vi "101_VI_Analysis_G-CLI.vi"() -> ()   [LabVIEW 2023]
doc: "This example uses the advanced VI Analyzer VIs to perform an analysis on an LLB of VIs. The \"New Task\" VI uses preset test settings loaded from a CFG file that was created from the VI Analyzer user interface. Certain advanced VIs are used to perform tasks like adding an LLB to the analysis, removing a single VI from the analysis, removing certain tests from the analysis, and modifying a configuration value on one test. Once the analysis performed by \"VIAn Run.vi\" is complete, the \"VIAn Easy Report.vi\" saves the analysis results to an HTML report."
uses:
  <vilib>/addons/analyzer/NI_VIAnalyzerTKVIs.lvlib
  <vilib>/Wiresmith Technology/G CLI/CLI Class/CLI.lvclass
panel:
  out "Custom Parameters":string[](array[string])
  out "VI in Analysis":string
  out "Analysis Progress":dbl(slide) scale=0.0..100.0
  out "Tests Run":string[](array[string])
  out "VIs Tested":path[](array[path])
  # "Overview: Demonstrates the use of the VI Analyzer and VI Analyzer Utility VIs to customize a programmatic analysis.\nRequirements: VI Analyzer Toolkit\nInstructions:\nRun the VI."
  # "Exclude these tests from the VI Analyzer Task."
  # "Set these tests to have 10 maximum failures for the VI Analyzer Task."
  # "Remove the top-level placeholder VI from the analysis."
  # "Disable the option on the \"VI Documentation\" test to analyze control descriptions."
  # "Show the progress of the analysis."
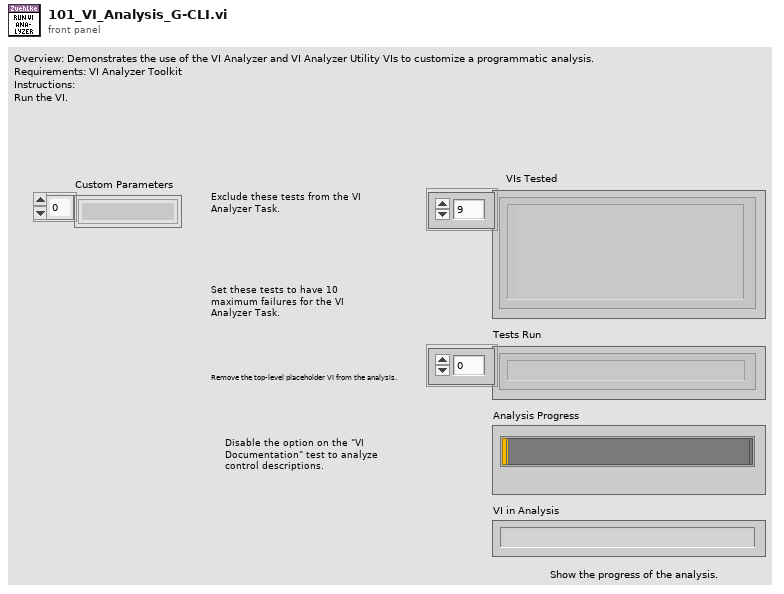
[diagram p1: front panel]
types:
  T1 = typedef "VIAnAPI Ref.ctl" = refnum<k1>
  T2 = typedef "VIAnCtl Results.ctl" = cluster{"Test Name":string, "Results Data":T3[], "Status":T4, "Exceed Max Fails?":bool}
  T3 = typedef "VIAnCtl ResultsData (index).ctl" = cluster{"Result Message":string, "Ref Index":i32}
  T4 = typedef "VIAnCtl ResultStatus.ctl" = enum16{"Pass", "Fail", "Skipped", "VI not loadable", "Test not loadable", "Test not runnable", "Test error out"}
  T5 = typedef "VIAnRes Parsed Results Data (by VI).ctl" = cluster{"VI Path":path, "Pass":cluster{"row":i32, "column":i32}[], "Fail":cluster{"row":i32, "column":i32}[], "Skipped":cluster{"row":i32, "column":i32}[], "VI not loadable":cluster{"row":i32, "column":i32}[], "Test not loadable":cluster{"row":i32, "column":i32}[], "Test not runnable":cluster{"row":i32, "column":i32}[], "Test error out":cluster{"row":i32, "column":i32}[]}
  T6 = typedef "VIAnRes Parsed Results Data (by Test).ctl" = cluster{"Test Name":string, "Pass":cluster{"VI Path":path, "index":cluster{"row":i32, "column":i32}}[], "Fail":cluster{"VI Path":path, "index":cluster{"row":i32, "column":i32}}[], "Skipped":cluster{"VI Path":path, "index":cluster{"row":i32, "column":i32}}[]}
  T7 = typedef "VIAnCtl Test Config Data.ctl" = cluster{"Test Name":string, "Config Ref":refnum<vi>, "Ref Valid?":bool, "Test Ranking":T8, "Max Failures":u32, "Test Path":path, "Control Values":T9[], "Selected?":bool}
  T8 = typedef "VIAnCtl TestRanking.ctl" = u16
  T9 = typedef "VIAnCtl Config Control Value.ctl" = cluster{"Control Name":string, "Control Value":variant}
  T10 = cluster{"Raw Results":T2[][], "Parsed Results Data (by VI)":T5[], "Parsed Results Data (by Test)":T6[], "Summary Statistics":cluster{"Passed Tests":i32, "Failed Tests":i32, "Skipped Tests":i32, "VIs not loadable":i32, "Tests not loadable":i32, "Tests not runnable":i32, "Test error out":i32, "Start Time":u32, "Total Time (s)":dbl}, "Test Config Data":T7[]}
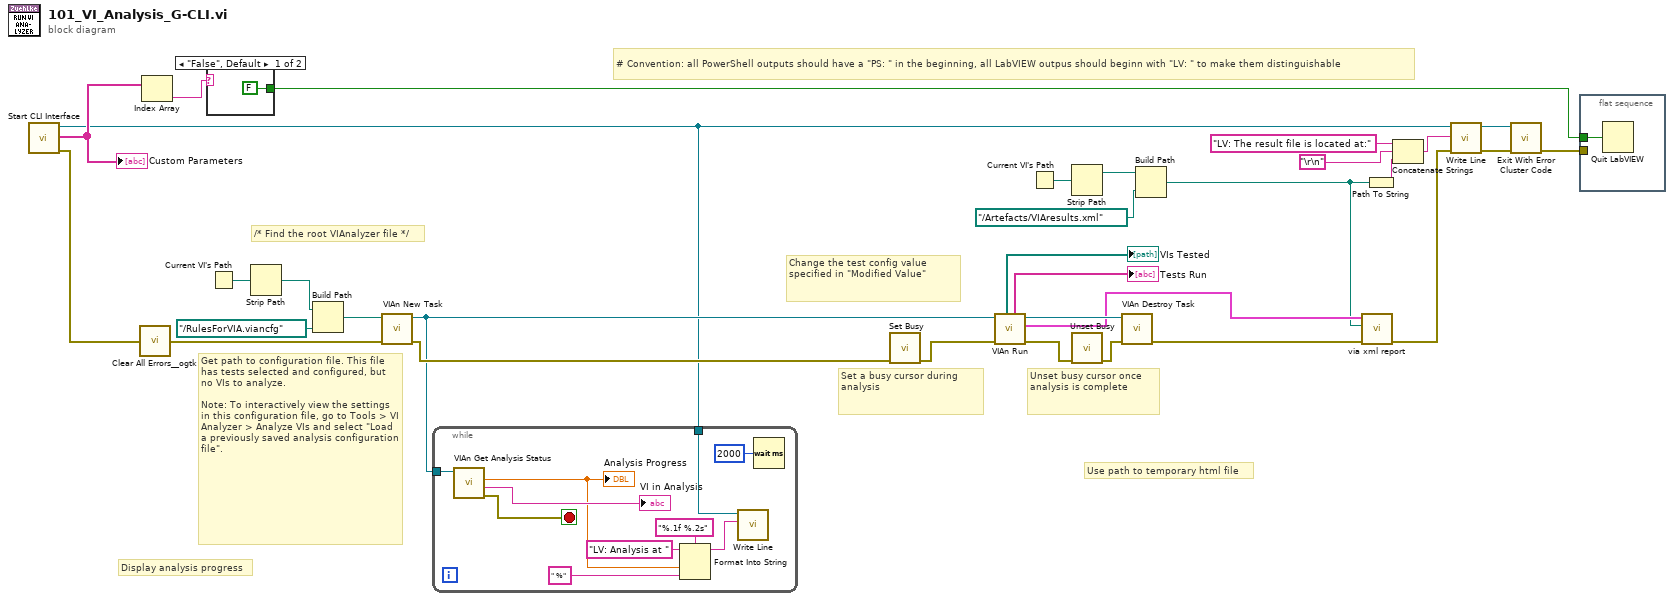
[diagram p0: block diagram]
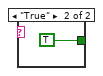
[diagram p2: hidden frame]
diagram:
  # "# Convention: all PowerShell outputs should have a \"PS: \" in the beginning, all LabVIEW outpus should beginn with \"LV: \" to make them distinguishable"
  # "/* Find the root VIAnalyzer file */"
  # "Display analysis progress"
  # "Unset busy cursor once analysis is complete"
  # "Set a busy cursor during analysis"
  # "Use path to temporary html file"
  # "Change the test config value specified in \"Modified Value\""
  # "Get path to configuration file. This file has tests selected and configured, but no VIs to analyze.\n\nNote: To interactively view the settings in this configuration file, go to Tools > VI Analyzer > Analyze VIs and select \"Load a previously saved analysis configuration file\"."
  n1 = call <vilib>:"Start CLI Interface.vi"() -> ("error out"=w15:errorcluster, "Custom Parameters"=w14:string[], "CLI out"=w10:refnum<class "CLI.lvclass">)  [unwired: 8 in, 1 out]
  "Custom Parameters" <- w14
  n2 = call <userlib>:"Clear All Errors__ogtk.vi"("Error In"=w15) -> ("Error Out"=w1:errorcluster)  [unwired: 3 in]
  n3 = Index Array(array=w14) -> (element=w12:string)  [unwired: 1 in]
  n4 = case shown="\"False\", Default" w12 {
    tunnel: [FALSE TRUE] -> w11
    frame "False", Default {
    }
    frame "True" {
    }
  }
  n5 = Current VI's Path() -> (path=w22:path)
  n6 = Strip Path(path=w22) -> (stripped path=w24:path)  [unwired: 1 out]
  n7 = Build Path(base path=w24, name or relative path=path "../RulesForVIA.viancfg" ("path")) -> (appended path=w21:path)
  n8 = call <vilib>:"VIAn New Task.vi"("error in (no error)"=w1, "Path to Configuration File"=w21) -> ("error out"=w32:errorcluster, "VI Analyzer Task"=w25:T1)  [unwired: 1 in, 7 out]
  n9 = while {
    tunnel: w25 -> [w44]
    tunnel: w10 -> [w40]
    stop <- w41 stop-if-true
    n10 = call <vilib>:"VIAn Get Analysis Status.vi"("VI Analyzer Task in"=w44) -> ("error out"=w41:errorcluster, "VI in Analysis"=→"VI in Analysis":string, "Percent Complete"=w39:dbl)  [unwired: 1 in, 7 out]
    "Analysis Progress" <- w39
    n11 = Format Into String(format string="%.1f %.2s", initial string="LV: Analysis at ", w39, " %" ("initial string")) -> (resulting string=w36:string)  [unwired: 1 in, 1 out]
    n12 = call <vilib>:"Write Line.vi"("Text to Write"=w36, "CLI in"=w40) -> ()  [unwired: 8 in, 2 out]
    n13 = Wait (ms)(milliseconds to wait=u32 2000) -> ()  [unwired: 1 out]
  }
  n14 = call <vilib>:"Set Busy.vi"("error in (no error)"=w32) -> ("error out"=w28:errorcluster)  [unwired: 3 in, 7 out]
  n15 = call <vilib>:"VIAn Run.vi"("error in (no error)"=w28, "VI Analyzer Task in"=w25) -> ("error out"=w27:errorcluster, "Analysis Results"=w16:T10, "VI Analyzer Task out"=w31:T1, "Tests Run"=→"Tests Run":string[], "VIs Tested"=→"VIs Tested":path[])  [unwired: 5 out]
  n16 = Current VI's Path() -> (path=w19:path)
  n17 = Strip Path(path=w19) -> (stripped path=w20:path)  [unwired: 1 out]
  n18 = call <vilib>:"Unset Busy.vi"("error in (no error)"=w27) -> ("error out"=w26:errorcluster)  [unwired: 1 in, 9 out]
  n19 = call <vilib>:"VIAn Destroy Task.vi"("error in (no error)"=w26, "VI Analyzer Task in"=w31) -> ("error out"=w17:errorcluster)  [unwired: 9 out]
  n20 = Build Path(base path=w20, name or relative path=path "../Artefacts/VIAresults.xml" ("path")) -> (appended path=w4:path)
  n21 = call <vilib>:"via xml report.vi"("error in (no error)"=w17, "Path"=w4, "Analysis Results"=w16) -> ("error out"=w8:errorcluster)  [unwired: 8 in]
  n22 = Path To String(path=w4) -> (string=w5:string)
  n23 = Concatenate Strings("LV: The result file is located at:" ("string"), "\r\n", w5) -> (w3:string)
  n24 = call <vilib>:"Write Line.vi"("error in (no error)"=w8, "Text to Write"=w3, "CLI in"=w10) -> ("error out"=w2:errorcluster, "CLI out"=w9:refnum<class "CLI.lvclass">)  [unwired: 7 in]
  n25 = call <vilib>:"Exit With Error Cluster Code.vi"("error in (no error)"=w2, "CLI in"=w9) -> ("error out"=w13:errorcluster)  [unwired: 9 in]
  n26 = flat-sequence {
    tunnel: w13 -> [_]
    tunnel: w11 -> [w45]
    frame #0 {
      n27 = Quit LabVIEW(quit? (T)=w45) -> ()
    }
  }
